vi "GoTo.vi"(6 "Busy":refnum<vi>, 8 "error in (no error)":errorcluster, 10 "Param":string, 11 "QuickSilver in":refnum<class "QuickSilver.lvclass">) -> (0 "error out":errorcluster, 2 "Response":string, 3 "QuickSilver out":refnum<class "QuickSilver.lvclass">)   [LabVIEW 2018, in "QuickSilver.lvclass"]
uses:
  QuickSilver.lvclass
  QuickSilver.lvclass/QuickSilver.ctl
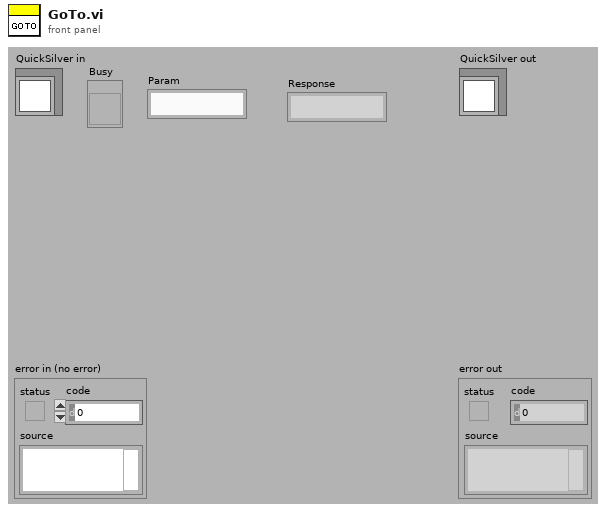
[diagram p1: front panel]
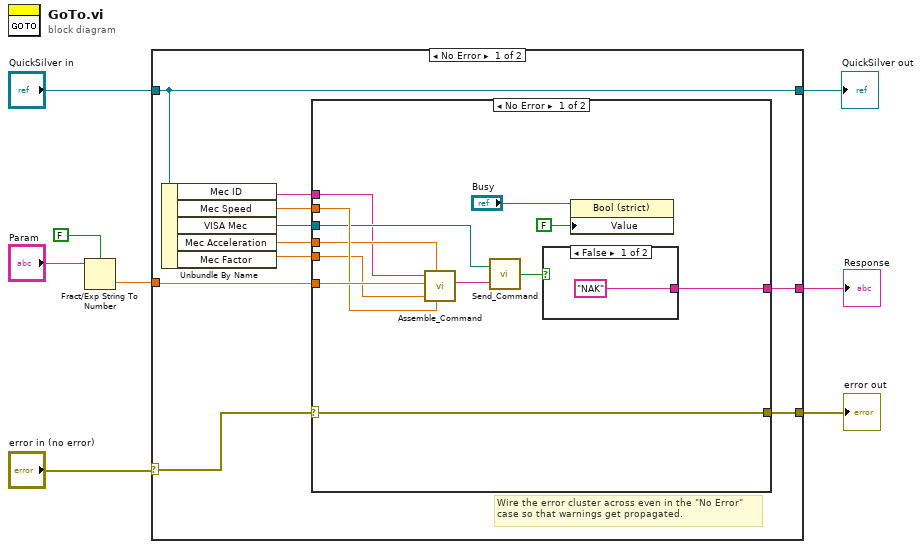
[diagram p0: block diagram]
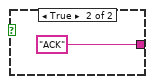
[diagram p2: hidden frame]
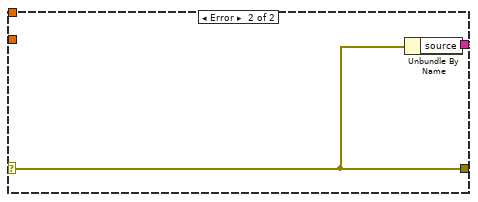
[diagram p3: hidden frame]
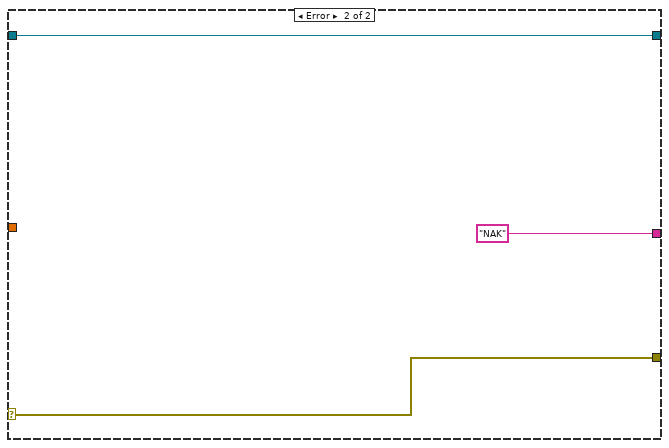
[diagram p4: hidden frame]
diagram:
  n1 = Fract/Exp String To Number(use system decimal point (T)=FALSE, string="Param") -> (number=w3:dbl)  [unwired: 3 out]
  n2 = case shown="No Error" "error in (no error)" {
    selector: "error in (no error)" -> [w15 w37]
    tunnel: [w18 w37] -> w6
    tunnel: [w14 w36] -> w4
    tunnel: "QuickSilver in" -> [w14 w36]
    tunnel: [w17 "NAK"] -> w5
    tunnel: w3 -> [w16 _]
    frame No Error {
      # "Wire the error cluster across even in the \"No Error\"\ncase so that warnings get propagated."
      n3 = Unbundle By Name(w14) -> ("Mec ID"=w13:string, "Mec Speed"=w12:dbl, "VISA Mec"=w11:refnum<visa-resource-name>, "Mec Acceleration"=w10:dbl, "Mec Factor"=w9:dbl)
      n4 = case shown="No Error" w15 {
        selector: w15 -> [w19 w34]
        tunnel: [w19 w34] -> w18
        tunnel: [w29 w33] -> w17
        tunnel: w16 -> [w28 _]
        tunnel: w12 -> [w27 _]
        tunnel: w10 -> [w26 _]
        tunnel: w11 -> [w25 _]
        tunnel: w13 -> [w24 _]
        tunnel: w9 -> [w23 _]
        frame No Error {
          n5 = call "Assemble_Command.vi"("Controller ID"=w24, "Acceleration"=w26, "Target"=w28, "Step factor"=w23, "Speed"=w27) -> ("command"=w30:string)  [unwired: 2 in, 3 out]
          n6 = call "Send_Command.vi"("write buffer"=w30, "VISA resource name"=w25) -> ("Command sent"=w21:bool)
          n7 = case shown="False" w21 {
            tunnel: ["NAK" "ACK"] -> w29
            frame False {
            }
            frame True {
            }
          }
          n8 = property class="Bool (strict)"(reference="Busy", "Value"=FALSE) -> ()  [unwired: 1 in, 2 out]
        }
        frame Error {
          n9 = Unbundle By Name(w34) -> ("source"=w33:string)
        }
      }
    }
    frame Error {
    }
  }
  "error out" <- w6
  "QuickSilver out" <- w4
  "Response" <- w5
